vi "Dynamic Saturation.vi"(11 "Voltage":dbl) -> (3 "Saturation Voltage":dbl)   [LabVIEW 2017]
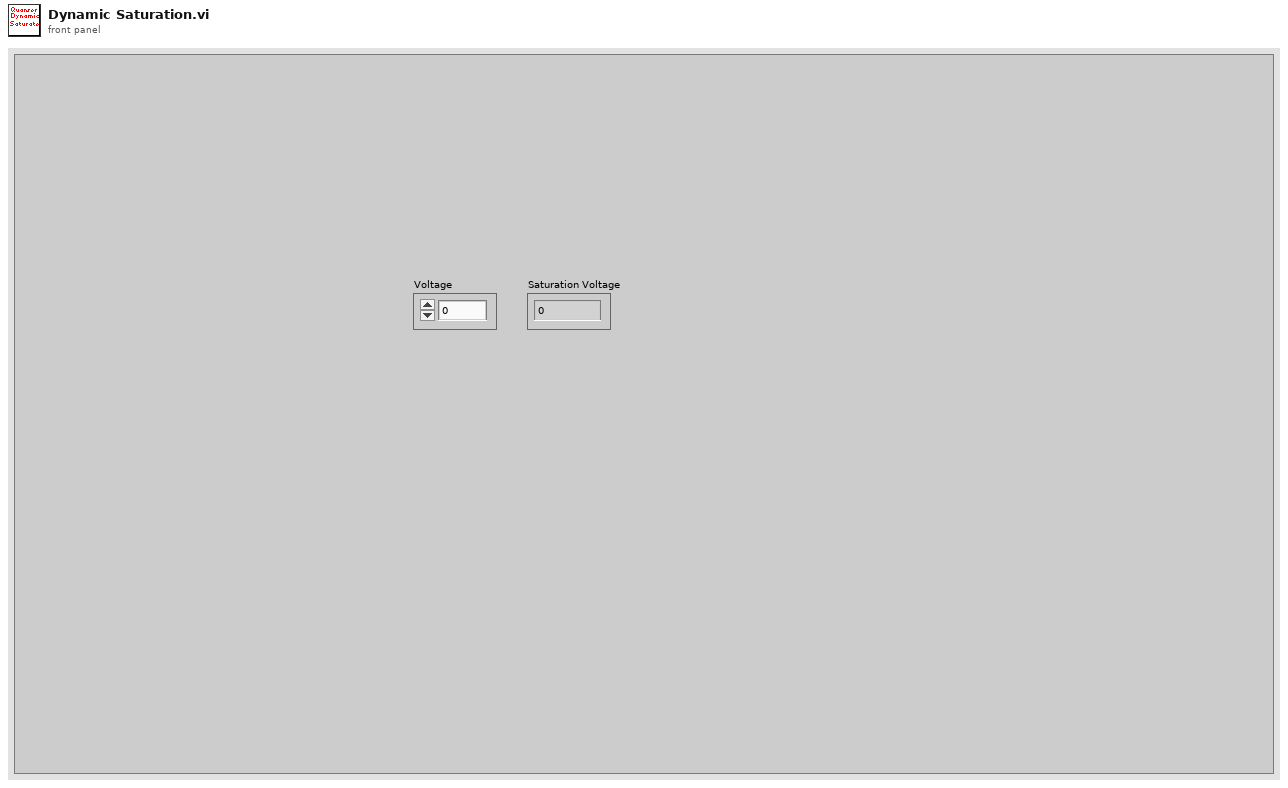
[diagram p1: front panel]
types:
  T1 = enum16{"Cooling off", "Heating up", "HOT! COOL IT", "normal operation"}
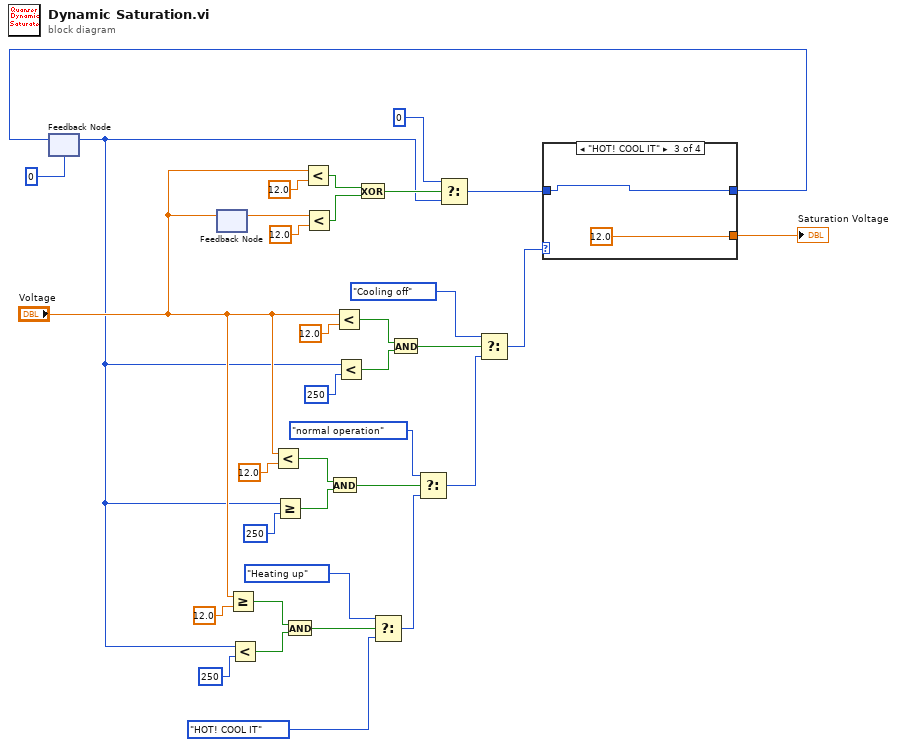
[diagram p0: block diagram]
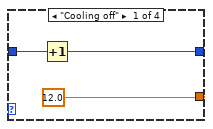
[diagram p2: hidden frame]
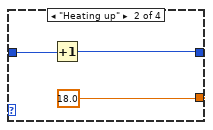
[diagram p3: hidden frame]
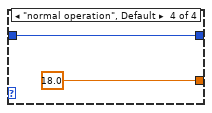
[diagram p4: hidden frame]
diagram:
  n1 = feedback #1(0) -> (w3:i32)
  n2 = feedback #2() -> (w7:dbl)  [unwired: 1 in]
  n3 = feedback-in #2("Voltage") -> ()
  n4 = Greater Or Equal?(x="Voltage", y=12.0) -> (x >= y?=w20:bool)
  n5 = Less?(x=w3, y=250) -> (x < y?=w19:bool)
  n6 = Less?(x="Voltage", y=12.0) -> (x < y?=w27:bool)
  n7 = Greater Or Equal?(x=w3, y=250) -> (x >= y?=w26:bool)
  n8 = And(x=w20, y=w19) -> (x .and. y?=w18:bool)
  n9 = Less?(x="Voltage", y=12.0) -> (x < y?=w6:bool)
  n10 = Less?(x=w7, y=12.0) -> (x < y?=w5:bool)
  n11 = And(x=w27, y=w26) -> (x .and. y?=w25:bool)
  n12 = Less?(x="Voltage", y=12.0) -> (x < y?=w33:bool)
  n13 = Less?(x=w3, y=250) -> (x < y?=w32:bool)
  n14 = Exclusive Or(1:w5, 2:w6) -> (0:w4:bool)
  n15 = Select(t=T1."Heating up", s=w18, f=T1."HOT! COOL IT") -> (s? t:f=w11:T1)
  n16 = And(x=w33, y=w32) -> (x .and. y?=w31:bool)
  n17 = Select(t=T1."normal operation", s=w25, f=w11) -> (s? t:f=w23:T1)
  n18 = Select(t=0, s=w4, f=w3) -> (s? t:f=w1:i32)
  n19 = Select(t=T1."Cooling off", s=w31, f=w23) -> (s? t:f=w15:T1)
  n20 = case shown="\"HOT! COOL IT\"" w15 {
    tunnel: [12.0 18.0 12.0 18.0] -> w14
    tunnel: w1 -> [w37 w40 w42 w44]
    tunnel: [w36 w39 w42 w44] -> w12
    frame "Cooling off" {
      n21 = Increment(x=w37) -> (x+1=w36:i32)
    }
    frame "Heating up" {
      n22 = Increment(x=w40) -> (x+1=w39:i32)
    }
    frame "HOT! COOL IT" {
    }
    frame "normal operation", Default {
    }
  }
  "Saturation Voltage" <- w14
  n23 = feedback-in #1(w12) -> ()
